vi "Write gplugin.vi"(0 "configuration":T1, 5 "Path":path=path "D:/EXP/ABC/ABC.gplugindata", 11 "error in":errorcluster) -> (15 "error out":errorcluster)   [LabVIEW 2021, in "InstrumentStudio Plug-In Editor.lvlib"]
uses:
  InstrumentStudio Plug-In Editor.lvlib
  controls/Data Holder.ctl
  <vilib>/xml/Load XML String.vi
  <vilib>/xml/Close Reference(Node).vi
  <vilib>/xml/NI_XML.lvlib
  <resource>/objmgr/DOMUserDefRef.rc
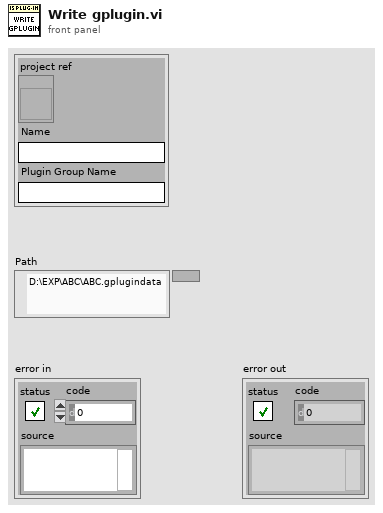
[diagram p1: front panel]
types:
  T1 = typedef "InstrumentStudio Plug-In Editor.lvlib/Data Holder.ctl" = cluster{"project ref":refnum<vi>, "Name":string, "Plugin Group Name":string}
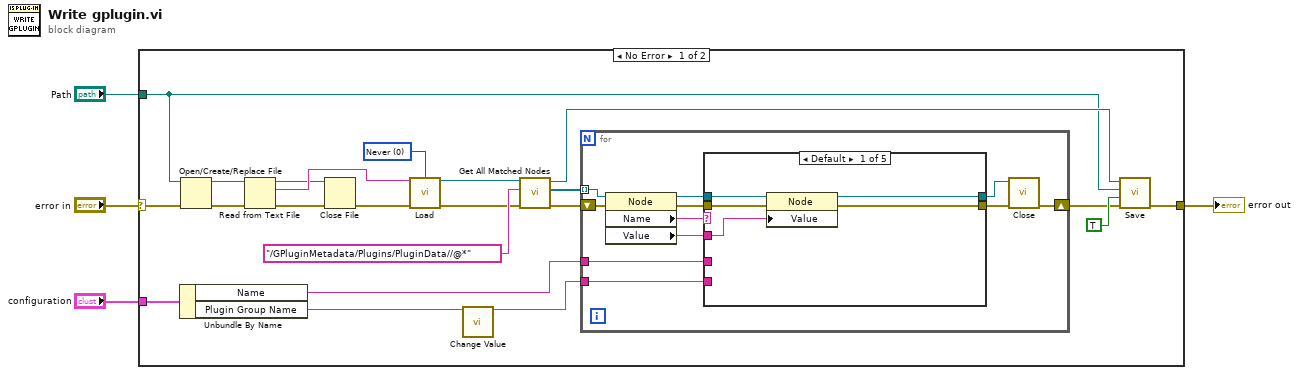
[diagram p0: block diagram]
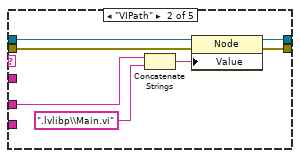
[diagram p2: hidden frame]
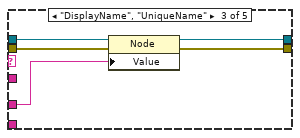
[diagram p3: hidden frame]
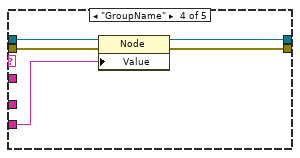
[diagram p4: hidden frame]
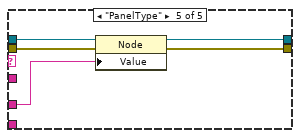
[diagram p5: hidden frame]
diagram:
  n1 = case shown="No Error" "error in" {
    selector: "error in" -> [w11 w65]
    tunnel: [w19 w65] -> w4
    tunnel: "Path" -> [w7 _]
    tunnel: "configuration" -> [w18 _]
    frame No Error {
      w24 = 0 items=["Never", "Always", "Auto"] ("validate on load (Auto)")
      n2 = Unbundle By Name(w18) -> ("Name"=w17:string, "Plugin Group Name"=w6:string)
      n3 = Open/Create/Replace File(file path (use dialog)=w7, error in=w11) -> (refnum out=w26:refnum<file>, error out=w10:errorcluster)  [unwired: 4 in, 1 out]
      n4 = Read from Text File(file (use dialog)=w26, error in=w10) -> (refnum out=w21:refnum<file>, text=w25:string, error out=w9:errorcluster)  [unwired: 2 in, 1 out]
      n5 = Close File(refnum=w21, error in=w9) -> (error out=w8:errorcluster)  [unwired: 1 out]
      n6 = call-poly <vilib>:"Load.vi"("XML string"=w25, "validate on load (Auto)"=w24, "error in (no error)"=w8) -> ("DOM document out"=w5:refnum<k20>, "error out"=w14:errorcluster)  [unwired: 10 in, 1 out]
      n7 = call "Change Value.vi"("String"=w6) -> ("String Out"=w16:string)  [unwired: 14 in]
      n8 = call <vilib>:"Get All Matched Nodes.vi"("error in (no error)"=w14, "XPath expression"="/GPluginMetadata/Plugins/PluginData//@*", "node in"=w5) -> ("error out"=w13:errorcluster, "node result array"=w15:refnum<k20>[], "node out"=w20:refnum<k20>)  [unwired: 6 in]
      n9 = for {
        tunnel: w15 -> [w37] mode=indexing
        tunnel: w17 -> [w33]
        tunnel: w16 -> [w32]
        shift-right: [w27] -> w12
        shift-left: w13 -> [w30]
        n10 = property class="Node"(reference=w37, error in=w30) -> (reference out=w36:refnum<k20>, error out=w29:errorcluster, "Name"=w34:string, "Value"=w31:string)
        n11 = case shown="Default" w34 {
          tunnel: w36 -> [w42 w49 w54 w59 w64]
          tunnel: [w41 w48 w53 w55 w63] -> w35
          tunnel: [w40 w43 w52 w56 w62] -> w28
          tunnel: w33 -> [_ w47 w51 _ w61]
          tunnel: w32 -> [_ _ _ w58 _]
          tunnel: w31 -> [w39 _ _ _ _]
          tunnel: w29 -> [w38 w44 w50 w57 w60]
          frame Default {
            n12 = property class="Node"(reference=w42, error in=w38, "Value"=w39) -> (reference out=w41:refnum<k20>, error out=w40:errorcluster)
          }
          frame "VIPath" {
            n13 = Concatenate Strings(w47, ".lvlibp\\Main.vi" ("string")) -> (w46:string)
            n14 = property class="Node"(reference=w49, error in=w44, "Value"=w46) -> (reference out=w48:refnum<k20>, error out=w43:errorcluster)
          }
          frame "DisplayName", "UniqueName" {
            n15 = property class="Node"(reference=w54, error in=w50, "Value"=w51) -> (reference out=w53:refnum<k20>, error out=w52:errorcluster)
          }
          frame "GroupName" {
            n16 = property class="Node"(reference=w59, error in=w57, "Value"=w58) -> (reference out=w55:refnum<k20>, error out=w56:errorcluster)
          }
          frame "PanelType" {
            n17 = property class="Node"(reference=w64, error in=w60, "Value"=w61) -> (reference out=w63:refnum<k20>, error out=w62:errorcluster)
          }
        }
        n18 = call-poly <vilib>:"Close.vi"("error in (no error)"=w28, "node"=w35) -> ("error out"=w27:errorcluster)  [unwired: 7 in]
      }
      n19 = call <vilib>:"Save.vi"("error in (no error)"=w12, "overwrite file (True)"=TRUE, "XML file path"=w7, "DOM document in"=w20) -> ("error out"=w19:errorcluster)  [unwired: 5 in, 2 out]
    }
    frame Error {
    }
  }
  "error out" <- w4
